vi "MessageFGV.vi"(6 "Operation":enum16{"Start", "Message", "Stop", "Disconnect"}(ring)=enum."Message", 8 "error in (no error)":errorcluster, 9 "Timeout (ms)":i32=-1, 10 "Payload":string, 11 "Command":string) -> (0 "error out":errorcluster, 3 "Response":string)   [LabVIEW 2019, in "MicronTemplateAPIs.lvlib" / "MicronTemplateAPIs.lvclass"]
uses:
  MicronTemplateAPIs.lvclass
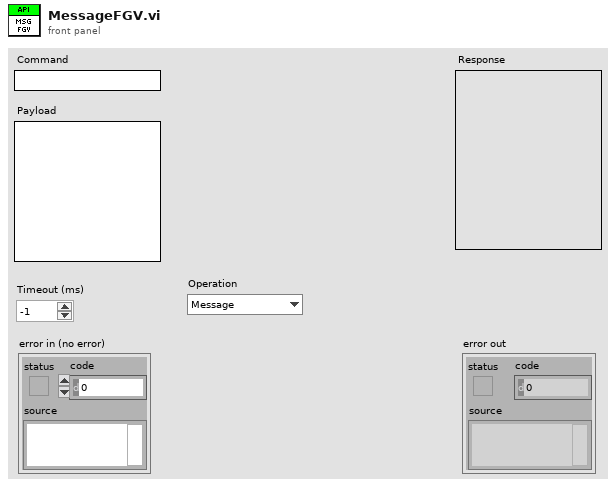
[diagram p1: front panel]
types:
  T1 = typedef "MicronClient.lvclass/ServiceDetails.ctl" = cluster{"MicronPath":path, "Network":string, "ServiceID":string, "Port":i32, "FullyQualifiedName":string, "UI":string, "Args":string, "Mode":string, "AutoRestartOnError?":bool, "Simulate?":bool}
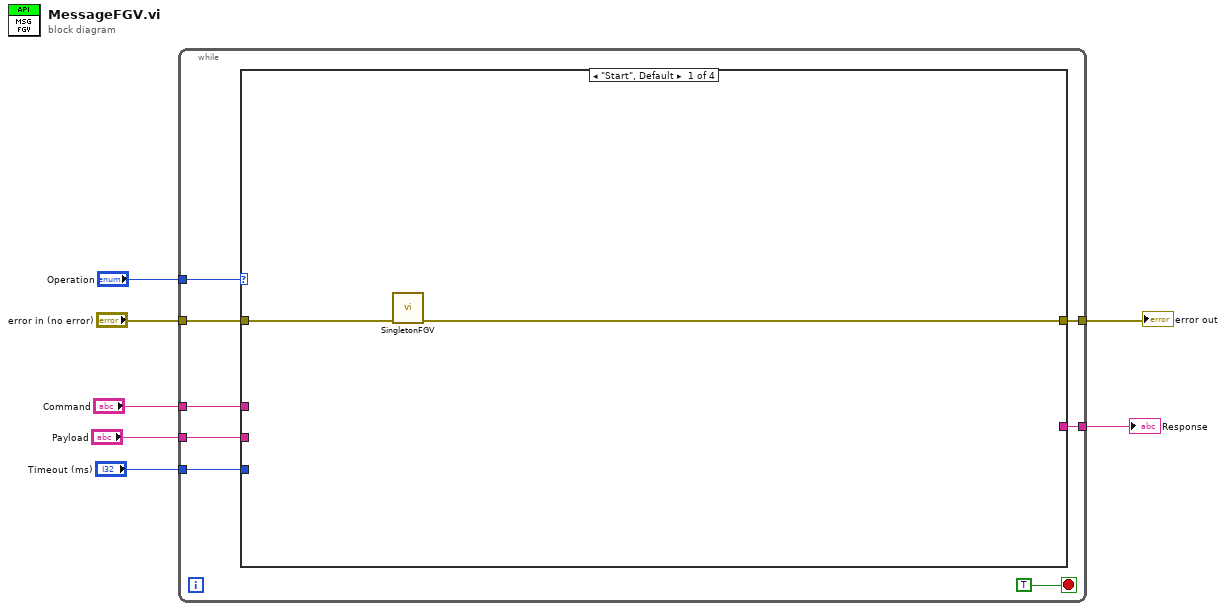
[diagram p0: block diagram]
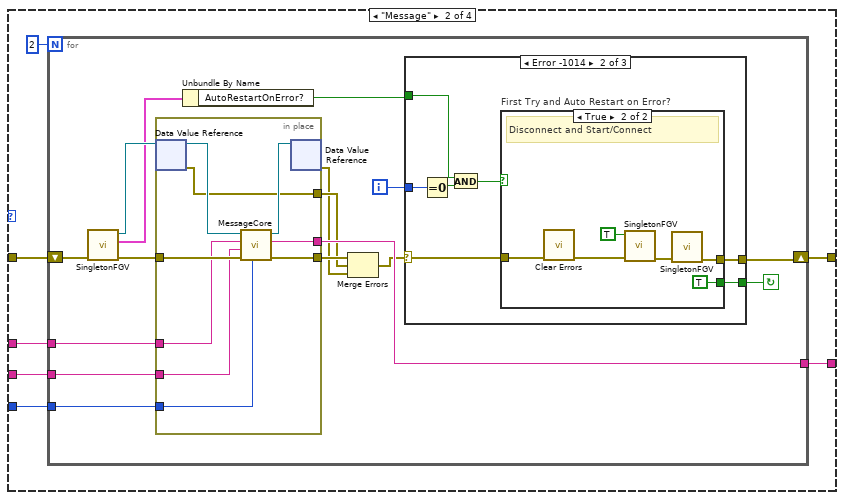
[diagram p2: hidden frame]
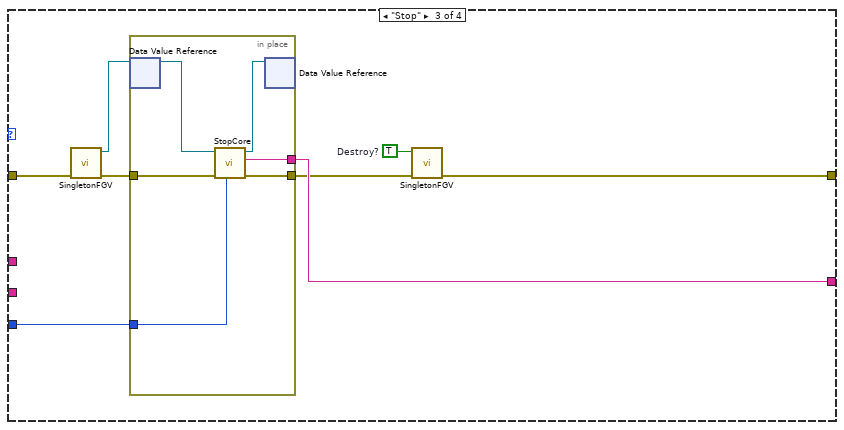
[diagram p6: hidden frame]
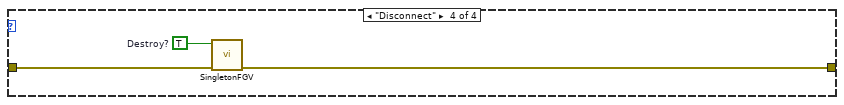
[diagram p7: hidden frame]
diagram:
  n1 = while {
    tunnel: "Operation" -> [w14]
    tunnel: "Command" -> [w13]
    tunnel: "Payload" -> [w12]
    tunnel: "Timeout (ms)" -> [w11]
    tunnel: "error in (no error)" -> [w10]
    tunnel: [w9] -> w6
    tunnel: [w8] -> w1
    stop <- TRUE stop-if-true
    n2 = case shown="\"Start\", Default" w14 {
      tunnel: w13 -> [_ w22 _ _]
      tunnel: w12 -> [_ w21 _ _]
      tunnel: w11 -> [_ w19 w66 _]
      tunnel: w10 -> [w17 w24 w73 w82]
      tunnel: [w16 w23 w68 w80] -> w9
      tunnel: [_ w20 w70 _] -> w8
      frame "Start", Default {
        n3 = call "SingletonFGV.vi"("error in (no error)"=w17) -> ("error out"=w16:errorcluster)  [unwired: 8 in, 2 out]
      }
      frame "Message" {
        n4 = for {
          N: 2 -> [_]
          tunnel: w21 -> [w36]
          tunnel: w19 -> [w34]
          shift-right: [w32] -> w23
          shift-left: w24 -> [w40]
          tunnel: w22 -> [w37]
          tunnel: [w35] -> w20
          i -> [w31]
          stop <- w30 continue-if-true
          n5 = call "SingletonFGV.vi"("error in (no error)"=w40) -> ("error out"=w39:errorcluster, "Connection Details"=w26:T1, "ServiceClientDVR"=w38:refnum<data-value>)  [unwired: 8 in]
          n6 = in-place {
            in-place-border: w39 -> [w65]
            in-place-border: [w64] -> w33
            in-place-border: w37 -> [w61]
            in-place-border: w36 -> [w60]
            in-place-border: [w59] -> w35
            in-place-border: w34 -> [w58]
            in-place-border: [w57] -> w28
            n7 = in-place-dvr #1(w38) -> (w63:refnum<class "MicronTemplateAPIs.lvclass">, w57:errorcluster)
            n8 = call-dynamic "MessageCore.vi"("Timeout (ms)"=w58, "error in (no error)"=w65, "Payload"=w60, "Command"=w61, "GRPCClient in"=w63) -> ("error out"=w64:errorcluster, "Response"=w59:string, "GRPCClient out"=w62:refnum<class "MicronTemplateAPIs.lvclass">)  [unwired: 4 in]
            n9 = in-place-dvr #1(w62) -> (w27:errorcluster)  [unwired: 1 out]
          }
          n10 = Unbundle By Name(w26) -> ("AutoRestartOnError?"=w25:bool)
          n11 = Merge Errors(w33, w28, w27) -> (w29:errorcluster)
          n12 = case shown="Error -1014" w29 {
            selector: w29 -> [w41 w48 w56]
            tunnel: [w41 w47 w56] -> w32
            tunnel: w25 -> [_ w44 _]
            tunnel: w31 -> [_ w46 _]
            tunnel: [_ w42 _] -> w30
            frame No Error {
            }
            frame Error {
              n13 = Equal To 0?(x=w46) -> (x = 0?=w45:bool)
              n14 = And(x=w44, y=w45) -> (x .and. y?=w43:bool)
              n15 = case "First Try and Auto Restart on Error?" shown="True" w43 {
                tunnel: w48 -> [w49 w55]
                tunnel: [w49 w52] -> w47
                tunnel: [_ TRUE] -> w42
                frame False {
                }
                frame True {
                  # "Disconnect and Start/Connect"
                  n16 = call <vilib>:"Clear Errors.vi"("error in (no error)"=w55) -> ("error out"=w51:errorcluster)  [unwired: 5 in, 1 out]
                  n17 = call "SingletonFGV.vi"("error in (no error)"=w51, "Destroy?"=TRUE) -> ("error out"=w53:errorcluster)  [unwired: 7 in, 2 out]
                  n18 = call "SingletonFGV.vi"("error in (no error)"=w53) -> ("error out"=w52:errorcluster)  [unwired: 8 in, 2 out]
                }
              }
            }
            frame Default {
              # "No Restart on any other error"
            }
          }
        }
      }
      frame "Stop" {
        w67 = TRUE  # Destroy?
        n19 = call "SingletonFGV.vi"("error in (no error)"=w73) -> ("error out"=w72:errorcluster, "ServiceClientDVR"=w71:refnum<data-value>)  [unwired: 8 in, 1 out]
        n20 = in-place {
          in-place-border: w72 -> [w79]
          in-place-border: [w78] -> w69
          in-place-border: [w75] -> w70
          in-place-border: w66 -> [w74]
          n21 = in-place-dvr #2(w71) -> (w77:refnum<class "MicronTemplateAPIs.lvclass">)  [unwired: 1 out]
          n22 = call-dynamic "StopCore.vi"("Timeout (ms)"=w74, "error in (no error)"=w79, "MicronGRPCClient in"=w77) -> ("error out"=w78:errorcluster, "Response"=w75:string, "MicronGRPCClient out"=w76:refnum<class "MicronTemplateAPIs.lvclass">)  [unwired: 6 in]
          n23 = in-place-dvr #2(w76) -> ()  [unwired: 2 out]
        }
        n24 = call "SingletonFGV.vi"("error in (no error)"=w69, "Destroy?"=w67) -> ("error out"=w68:errorcluster)  [unwired: 7 in, 2 out]
      }
      frame "Disconnect" {
        w81 = TRUE  # Destroy?
        n25 = call "SingletonFGV.vi"("error in (no error)"=w82, "Destroy?"=w81) -> ("error out"=w80:errorcluster)  [unwired: 7 in, 2 out]
      }
    }
  }
  "error out" <- w6
  "Response" <- w1
